vi "Project - broken.vi"() -> ()   [LabVIEW 2023]
uses:
  <instrlib>/Agilent N934X Series/Agilent N934X Series.lvlib
  <vilib>/Utility/file.llb/Read Delimited Spreadsheet (string).vi
  <instrlib>/Agilent N934X Series/Public/Configure/Configure Frequency (Start Stop).vi
  System.Windows.Forms
panel:
  out "Start Frequency (MHz)":dbl=5925.0
  out "Start Distance (ft)":dbl
  in  "Distance Unit (0: Meter)":i32(ring) items=["Meter", "Feet"]
  out "loop#":i32
  out "size(s)":i32
  out "Trace Data":dbl[](array[numeric])
  in  "Measurement Mode (0: Off)":i32(ring) items=["Off", "Channel Power Measurement", "Adjacent Channel Power Ratio Measurement", "Occupied Bandwidth Measurement", "Spectrum Monitor", "Spectrum Emission Mask", "Channel Scanner", "AM Measurement", "ASK Measurement", "FM Measurement", "FSK Measurement"]
  in  "Measurement Type (0: Spectrum Analyzer)":i32(ring) items=["Spectrum Analyzer", "Tracking Generator", "Power Meter", "Modulation Analyzer", "Reflection Measurement"]
  out "Instrument Firmware Revision":string
  out "Instrument Driver Revision":string
  in  "VISA resource name":refnum<visa-resource-name>
  in  "jkjk":bool
  out "jkjk":string
  out "jkjk":string
  out "jkjk":string
  in  "jkjk":bool
  in  "Tab Control":T1(tab)
  in  "?":bool
  out "?":string
  out "Step:":i32
  in  "IIM":bool
  out "Waveform Graph":dbl[](graph)
  in  "?":refnum<k24>(container)
  out "Section:":string
  in  "Stop Distance (ft)":dbl=0.15
  in  "Length of Cable (ft) 2":dbl
  in  "Cable Attenuation (dB/ft) 2":dbl
  in  "Velocity Factor (%) 2":dbl
  # "VSWR and Distance to Fault Test"
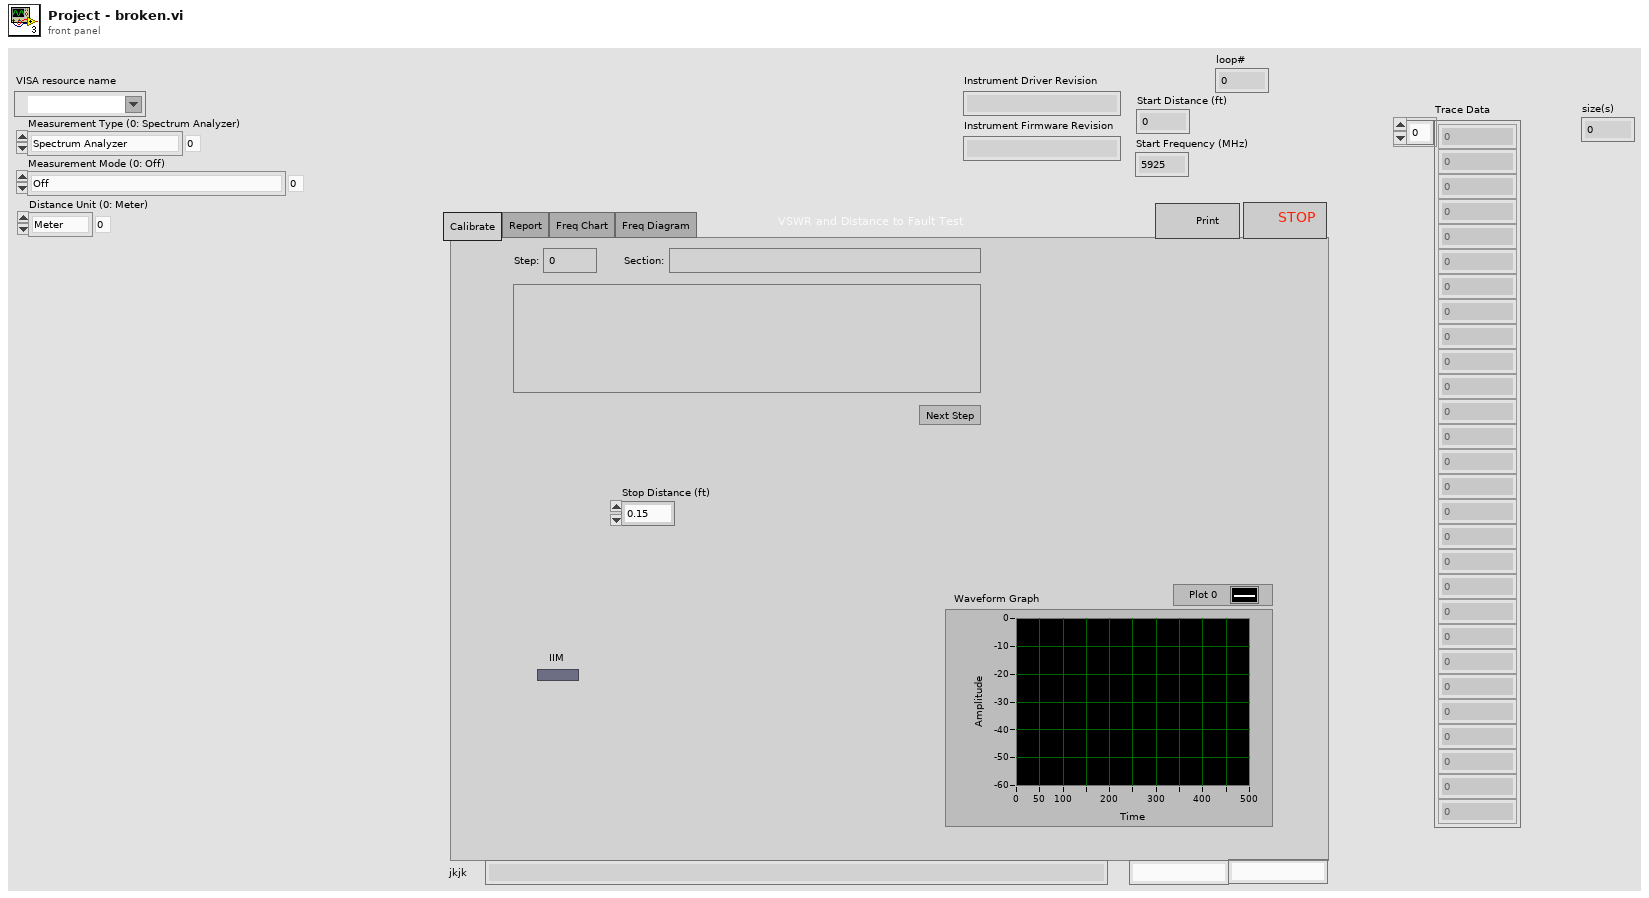
[diagram p1: front panel]
types:
  T1 = enum32{"Calibrate", "Report", "Freq Chart", "Freq Diagram"}
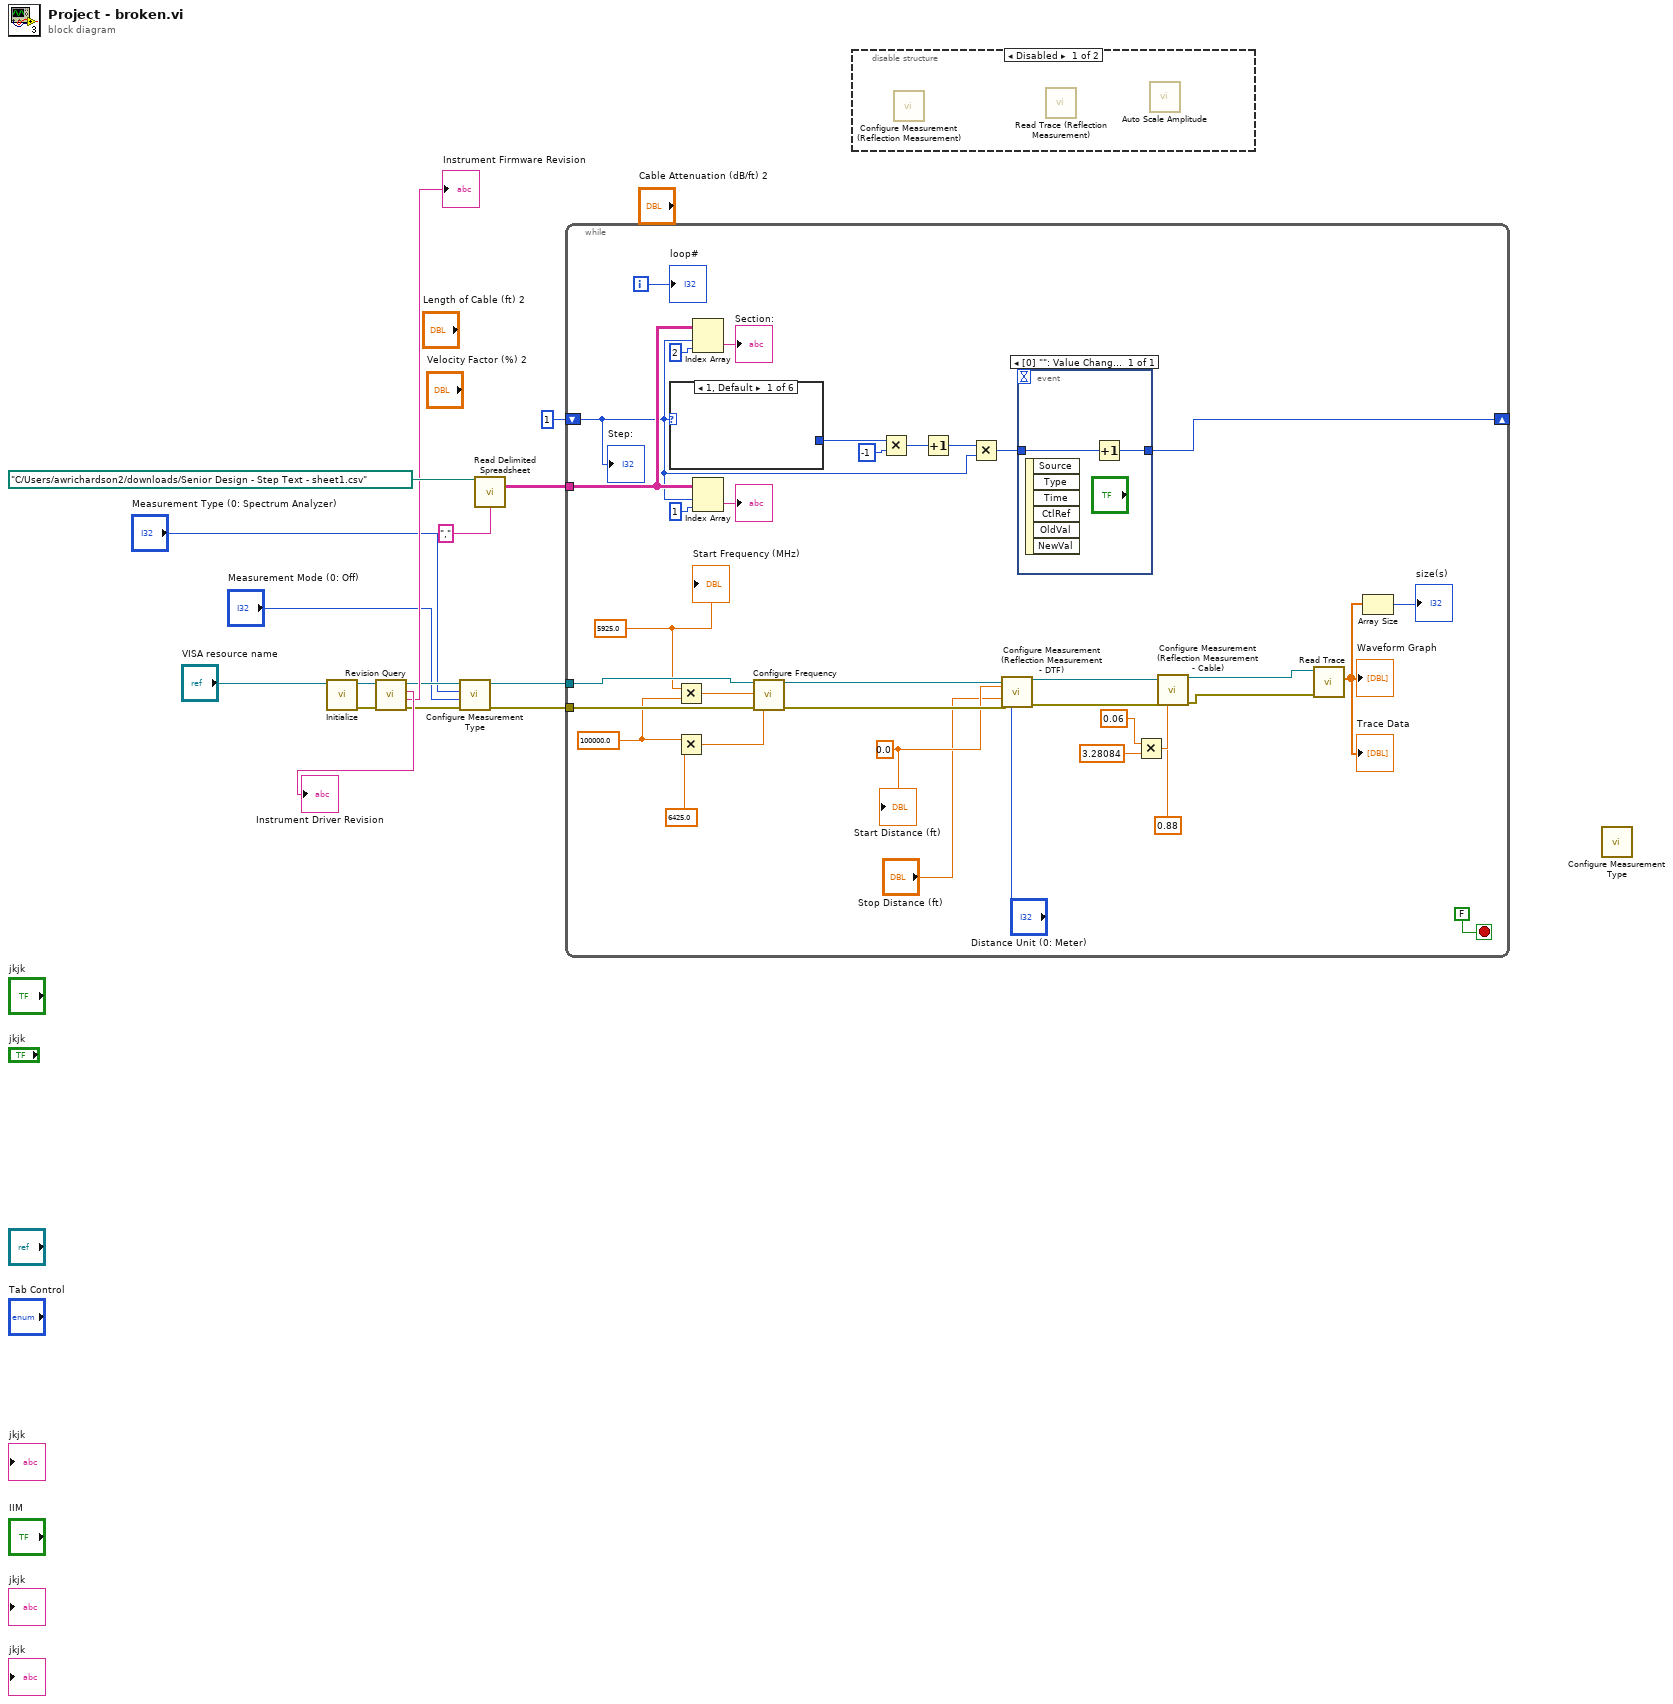
[diagram p0: block diagram]
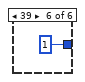
[diagram p7: hidden frame]
diagram:
  n1 = call <instrlib>:"Initialize.vi"("VISA resource name"="VISA resource name") -> ("error out"=w9:errorcluster, "VISA resource name out"=w10:refnum<visa-resource-name>)  [unwired: 9 in]
  n2 = call <instrlib>:"Revision Query.vi"("error in (no error)"=w9, "VISA resource name"=w10) -> ("error out"=w5:errorcluster, "Instrument Firmware Revision"=→"Instrument Firmware Revision":string, "Instrument Driver Revision"=→"Instrument Driver Revision":string, "VISA resource name out"=w6:refnum<visa-resource-name>)  [unwired: 6 in]
  n3 = call <instrlib>:"Configure Measurement Type.vi"("error in (no error)"=w5, "Measurement Mode (0: Off)"="Measurement Mode (0: Off)", "Measurement Type (0: Spectrum Analyzer)"="Measurement Type (0: Spectrum Analyzer)", "VISA resource name"=w6) -> ("error out"=w2:errorcluster, "VISA resource name out"=w1:refnum<visa-resource-name>)  [unwired: 6 in]
  n4 = call-poly <vilib>:"Read Delimited Spreadsheet.vi"("file path (dialog if empty)"=path "C:/Users/awrichardson2/downloads/Senior Design - Step Text - sheet1.csv", "delimiter (\\t)"="," ("delimiter (\\t)")) -> ("all rows"=w12:string[][])  [unwired: 8 in, 5 out]
  n5 = while {
    shift-right: [w49] -> _
    shift-left: 1 -> [w39]
    tunnel: w12 -> [w41]
    tunnel: w2 -> [w33]
    tunnel: w1 -> [w34]
    i -> [w36]
    stop <- FALSE stop-if-true
    w17 = 100000.0 ("y")
    w19 = 5925.0 ("Start Frequency (9E+3 Hz)")
    w21 = 0.0 ("Distance Start (0.12 meters)")
    n6 = case shown="1, Default" w39 {
      tunnel: [_ _ _ _ _ 1] -> w48
      frame 1, Default {
      }
      frame 2 {
      }
      frame 3 {
      }
      frame 4 {
      }
      frame 5 {
      }
      frame 39 {
      }
    }
    n7 = Multiply(x=w19, y=w17) -> (x*y=w18:dbl)
    n8 = Multiply(x=w17, y=6425.0) -> (x*y=w35:dbl)
    n9 = Index Array(array=w41, index (row)=w39, index (col)=2) -> (element=→"Section:":string)
    n10 = Index Array(array=w41, index (row)=w39, index (col)=1) -> (element=→"?":string)
    n11 = call-poly <instrlib>:"Configure Frequency.vi"("VISA resource name"=w34, "Start Frequency (9E+3 Hz)"=w18, "error in (no error)"=w33, "Stop Frequency (7E+9 Hz)"=w35) -> ("VISA resource name out"=w31:refnum<visa-resource-name>, "error out"=w30:errorcluster)  [unwired: 10 in]
    n12 = Multiply(x=w48, y=-1) -> (x*y=w46:i32)
    n13 = Increment(x=w46) -> (x+1=w45:i32)
    n14 = Multiply(x=w45, y=w39) -> (x*y=w50:i32)
    n15 = call <instrlib>:"Configure Measurement (Reflection Measurement - DTF).vi"("VISA resource name"=w31, "Distance Unit (0: Meter)"="Distance Unit (0: Meter)", "Distance Start (0.12 meters)"=w21, "Distance Stop (0.15 meter)"="Stop Distance (ft)", "error in (no error)"=w30) -> ("VISA resource name out"=w25:refnum<visa-resource-name>, "error out"=w24:errorcluster)  [unwired: 9 in]
    n16 = event shown="[0] \"\": Value Change" {
      selector: _ -> [_]
      dyn-events: _ -> [_]
      timeout: _ -> [_]
      tunnel: w50 -> [w54]
      tunnel: [w53] -> w49
      event Value Change {
        n17 = event-data() -> ()  [unwired: 1 in, 6 out]
        n18 = Increment(x=w54) -> (x+1=w53:i32)
      }
    }
    n19 = Multiply(x=0.06 ("Attenuation (0 dB/m)"), y=3.28084) -> (x*y=w27:dbl)
    n20 = call <instrlib>:"Configure Measurement (Reflection Measurement - Cable).vi"("VISA resource name"=w25, "Attenuation (0 dB/m)"=w27, "error in (no error)"=w24, "Velocity Factor (1.5)"=0.88) -> ("VISA resource name out"=w22:refnum<visa-resource-name>, "error out"=w23:errorcluster)  [unwired: 10 in]
    n21 = call <instrlib>:"Read Trace.vi"("error in (no error)"=w23, "VISA resource name"=w22) -> ("Trace Data"=w38:dbl[])  [unwired: 7 in, 2 out]
    "Waveform Graph" <- w38
    "Trace Data" <- w38
    n22 = Array Size(array=w38) -> (size(s)=→"size(s)":i32)
    "Step:" <- w39
    "loop#" <- w36
    "Start Distance (ft)" <- w21
    "Start Frequency (MHz)" <- w19
  }
  n23 = disable-structure shown="Disabled" {
    frame Disabled {
      n24 = call <instrlib>:"Configure Measurement (Reflection Measurement).vi"() -> ()  [unwired: 14 in, 2 out]
      n25 = call <instrlib>:"Read Trace (Reflection Measurement).vi"() -> ()  [unwired: 9 in, 3 out]
      n26 = call <instrlib>:"Auto Scale Amplitude.vi"() -> ()  [unwired: 10 in, 2 out]
    }
    frame Enabled {
    }
  }
  n27 = call <instrlib>:"Configure Measurement Type.vi"() -> ()  [unwired: 10 in, 2 out]
